vi "my Convert ROI to Point.vi"(7 "error in (no error)":errorcluster, 10 "ROI Descriptor":T2 {"Contours"."Type" items=["No Selection", "Point", "Line", "Rectangle", "Oval", "Polygon", "Freehand Region", "Annulus", "Unused2", "Unused3", "Broken Line", "Freehand Line", "Rotated Rectangle"]}) -> (0 "error out":errorcluster, 1 "Is a Point?":bool, 3 "Point":T1 {"Y" format="%.2f"; "X" format="%.2f"})   [LabVIEW 2021, in "Image.lvlib"]
doc: "Converts an ROI Descriptor to a point element."
uses:
  Image.lvlib
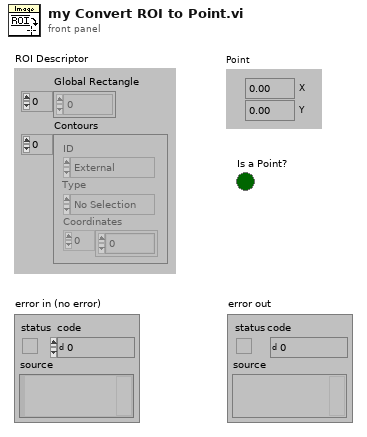
[diagram p1: front panel]
types:
  T1 = typedef "IMAQ Point" = cluster{"X":sgl, "Y":sgl}
  T2 = typedef "ROI Descriptor" = cluster{"Global Rectangle":i32[], "Contours":cluster{"ID":enum32{"External", "Internal"}, "Type":u32, "Coordinates":i32[]}[]}
  T3 = cluster{"ID":enum32{"External", "Internal"}, "Type":u32, "Coordinates":i32[]}[]
  T4 = cluster{"ID":enum32{"External", "Internal"}, "Type":u32, "Coordinates":i32[]}
  T5 = cluster{"Coordinates[0]":i32, "Coordinates[1]":i32}
  T6 = cluster{"Coordinates[0]":sgl, "Coordinates[1]":sgl}
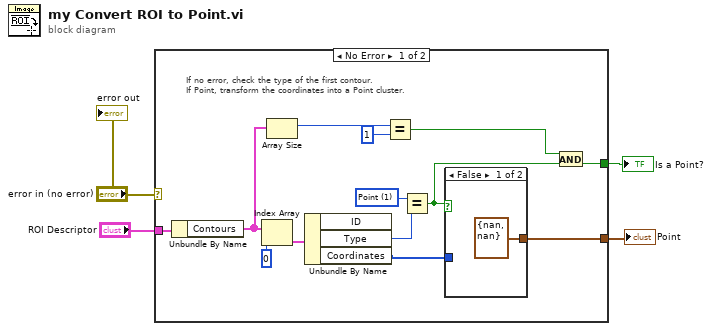
[diagram p0: block diagram]
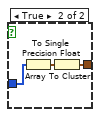
[diagram p2: hidden frame]
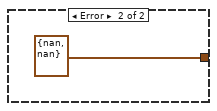
[diagram p3: hidden frame]
diagram:
  n1 = case shown="No Error" "error in (no error)" {
    tunnel: [w12 T1 {"X"=nan, "Y"=nan} ("Point")] -> w4
    tunnel: "ROI Descriptor" -> [w11 _]
    tunnel: [w6 _] -> w1
    frame No Error {
      w14 = u32 1 items=["No Selection", "Point", "Line", "Rectangle", "Oval", "Polygon", "Free", "Annulus", "Unused2", "Unused3", "Broken Line", "Free Hand Line", "Rotated Rectangle"] ("Type")
      # "If no error, check the type of the first contour.\nIf Point, transform the coordinates into a Point cluster."
      n2 = Unbundle By Name(w11) -> ("Contours"=w9:T3)
      n3 = Index Array(array=w9, index=0 ("Index")) -> (element=w16:T4)
      n4 = Array Size(array=w9) -> (size(s)=w8:i32)
      n5 = Unbundle By Name(w16) -> ("Type"=w13:u32, "Coordinates"=w15:i32[])  [unwired: 1 out]
      n6 = Equal?(x=w8, y=1) -> (x = y?=w5:bool)
      n7 = Equal?(x=w14, y=w13) -> (x = y?=w10:bool)
      n8 = case shown="False" w10 {
        tunnel: w15 -> [_ w21]
        tunnel: [T1 {"X"=nan, "Y"=nan} ("Point") w19] -> w12
        frame False {
        }
        frame True {
          n9 = Array To Cluster(array=w21) -> (cluster=w20:T5)
          n10 = To Single Precision Float(number=w20) -> (single precision float=w19:T6)
        }
      }
      n11 = And(x=w5, y=w10) -> (x .and. y?=w6:bool)
    }
    frame Error {
    }
  }
  "Point" <- w4
  "Is a Point?" <- w1
  "error out" <- "error in (no error)"
